vi "马里奥动图.vi"() -> ()   [LabVIEW 2018]
panel:
  out "布尔":bool
  out "滑动杆":dbl(slide) scale=0.0..10.0
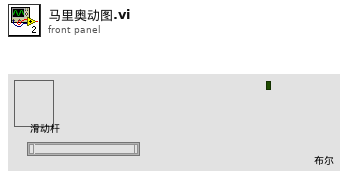
[diagram p1: front panel]
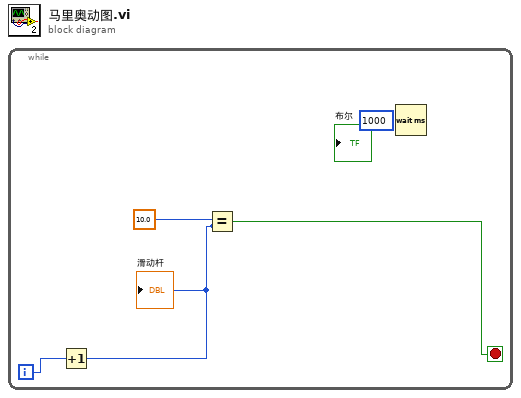
[diagram p0: block diagram]
diagram:
  n1 = while {
    i -> [w3]
    stop <- w2 stop-if-true
    w1 = 10.0 ("y")
    (unwired) u32 1000 ("毫秒计时值")
    n2 = Increment(x=w3) -> (x+1=w1:i32)
    "滑动杆" <- w1
    n3 = Equal?(y=w1) -> (x = y?=w2:bool)  [unwired: 1 in]
    n4 = Wait (ms)() -> ()  [unwired: 1 in, 1 out]
  }
